vi "S2DS_ConfigReadWC (SubVI).vi"(0 "Refnum in":T3, 1 "WC Info list (in)":T1, 2 "Update present value?":bool, 3 "error in (no error)":errorcluster) -> (6 "Refnum out":T3, 7 "WC Info list (out)":T1, 9 "error out":errorcluster)   [LabVIEW 2025]
uses:
  <vilib>/Utility/config.llb/Config Data RefNum.ctl
  TYPE DEFS/S2DS_WC info.ctl
  TYPE DEFS/S2DS_Single WC info.ctl
  <vilib>/Utility/config.llb/Read Key (U32).vi
  <vilib>/Utility/config.llb/Read Key (String).vi
  <vilib>/Utility/config.llb/Read Key (Double).vi
  <vilib>/Utility/config.llb/NI_LVConfig.lvlib
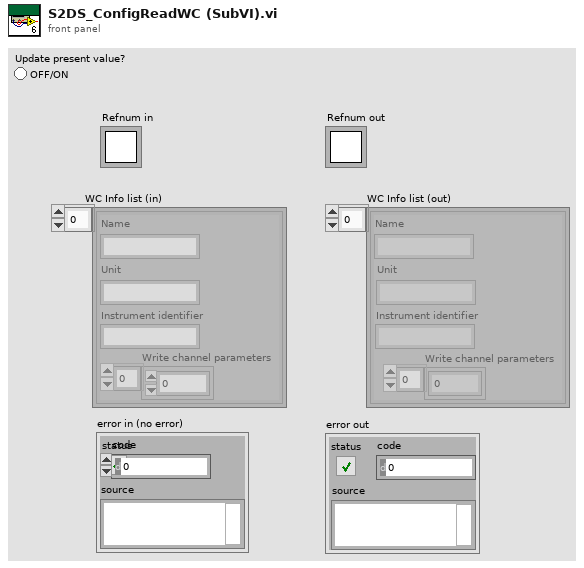
[diagram p1: front panel]
types:
  T1 = typedef "S2DS_WC info.ctl" = T2[]
  T2 = typedef "S2DS_Single WC info.ctl" = cluster{"Instrument identifier":string, "Write channel parameters":dbl[], "Name":string, "Unit":string}
  T3 = typedef "NI_LVConfig.lvlib/Config Data RefNum.ctl" = refnum<k1>
  T4 = cluster{"Instrument identifier":string, "Write channel parameters":dbl[], "Name":string, "Unit":string}
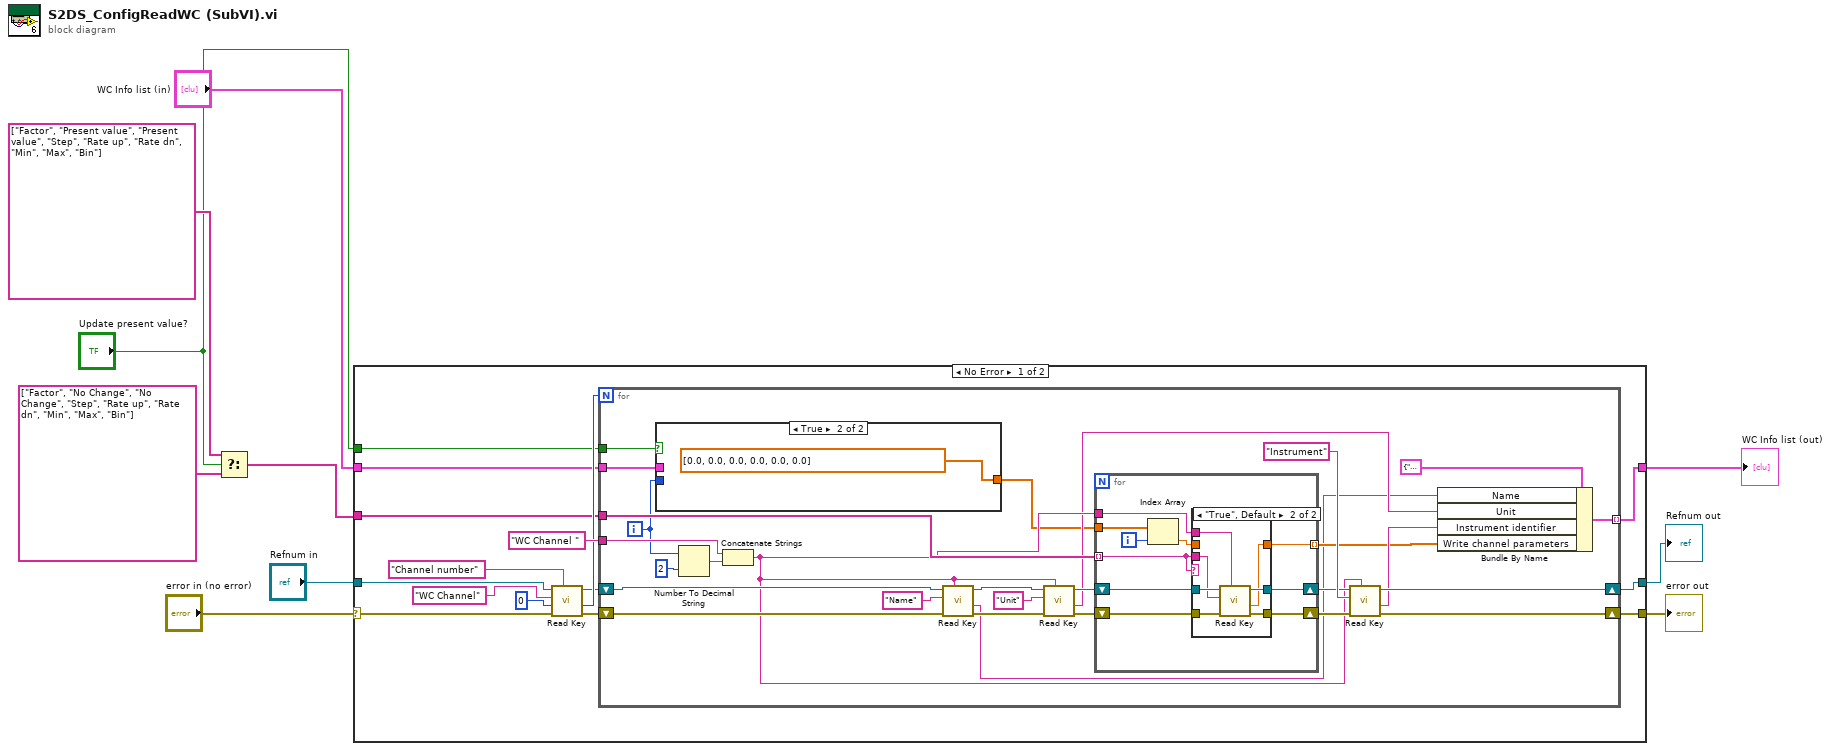
[diagram p0: block diagram]
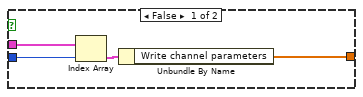
[diagram p2: hidden frame]
diagram:
  n1 = Select(t=string[] ["Factor", "Present value", "Present value", "Step", "Rate up", "Rate dn", "Min", "Max", "Bin"], s="Update present value?", f=string[] ["Factor", "No Change", "No Change", "Step", "Rate up", "Rate dn", "Min", "Max", "Bin"]) -> (s? t:f=w3:string[])
  n2 = case shown="No Error" "error in (no error)" {
    selector: "error in (no error)" -> [w15 w80]
    tunnel: [w25 w80] -> w10
    tunnel: [w24 w79] -> w9
    tunnel: [w22 w81] -> w8
    tunnel: "WC Info list (in)" -> [w12 w81]
    tunnel: "Refnum in" -> [w14 w79]
    tunnel: w3 -> [w13 _]
    tunnel: "Update present value?" -> [w11 _]
    frame No Error {
      n3 = call-poly <vilib>:"Read Key.vi"("section"="Channel number", "error in (no error)"=w15, "default value"=u32 0, "key"="WC Channel", "refnum"=w14) -> ("error out"=w16:errorcluster, "value"=w18:u32, "refnum out"=w17:T3)  [unwired: 4 out]
      n4 = for {
        N: w18 -> [_]
        shift-right: [w41] -> w24
        shift-left: w17 -> [w53]
        shift-right: [w40] -> w25
        shift-left: w16 -> [w52]
        tunnel: "WC Channel " -> [w49]
        tunnel: w13 -> [w39]
        tunnel: [w33] -> w22 mode=indexing
        tunnel: w12 -> [w29]
        tunnel: w11 -> [w26]
        i -> [w28]
        n5 = case shown="True" w26 {
          tunnel: w29 -> [w57 _]
          tunnel: w28 -> [w56 _]
          tunnel: [w54 dbl[] [0.0, 0.0, 0.0, 0.0, 0.0, 0.0] ("Write channel parameters")] -> w27
          frame False {
            n6 = Index Array(array=w57, index=w56) -> (element=w55:T2)
            n7 = Unbundle By Name(w55) -> ("Write channel parameters"=w54:dbl[])
          }
          frame True {
          }
        }
        n8 = Number To Decimal String(number=w28, width (-)=i16 2) -> (decimal integer string=w51:string)
        n9 = Concatenate Strings(w49, w51) -> (w36:string)
        n10 = call-poly <vilib>:"Read Key.vi"("section"=w36, "error in (no error)"=w52, "key"="Name", "refnum"=w53) -> ("error out"=w46:errorcluster, "value"=w30:string, "refnum out"=w47:T3)  [unwired: 2 in, 3 out]
        n11 = call-poly <vilib>:"Read Key.vi"("section"=w36, "error in (no error)"=w46, "key"="Unit", "refnum"=w47) -> ("error out"=w44:errorcluster, "value"=w31:string, "refnum out"=w43:T3)  [unwired: 2 in, 3 out]
        n12 = for {
          tunnel: w39 -> [w62] mode=indexing
          shift-right: [w67] -> w37
          shift-left: w43 -> [w68]
          shift-right: [w63] -> w38
          shift-left: w44 -> [w66]
          tunnel: w36 -> [w65]
          tunnel: [w64] -> w34 mode=indexing
          tunnel: w27 -> [w61]
          i -> [w60]
          n13 = Index Array(array=w61, index=w60) -> (element=w59:dbl)
          n14 = case shown="\"True\", Default" w62 {
            tunnel: w68 -> [w70 w78]
            tunnel: [w70 w77] -> w67
            tunnel: w66 -> [w71 w76]
            tunnel: w65 -> [_ w75]
            tunnel: w62 -> [_ w74]
            tunnel: [w69 w73] -> w64
            tunnel: [w71 w72] -> w63
            tunnel: w59 -> [w69 _]
            frame "No Change" {
            }
            frame "True", Default {
              n15 = call-poly <vilib>:"Read Key.vi"("section"=w75, "error in (no error)"=w76, "key"=w74, "refnum"=w78) -> ("error out"=w72:errorcluster, "value"=w73:dbl, "refnum out"=w77:T3)  [unwired: 1 in, 4 out]
            }
          }
        }
        n16 = call-poly <vilib>:"Read Key.vi"("section"=w36, "error in (no error)"=w38, "key"="Instrument", "refnum"=w37) -> ("error out"=w40:errorcluster, "value"=w35:string, "refnum out"=w41:T3)  [unwired: 2 in, 3 out]
        n17 = Bundle By Name(cluster=T4 {"Instrument identifier"="", "Write channel parameters"=[], "Name"="", "Unit"=""} ("Write channel info"), "Name"=w30, "Unit"=w31, "Instrument identifier"=w35, "Write channel parameters"=w34) -> (w33:T4)
      }
    }
    frame Error {
    }
  }
  "error out" <- w10
  "Refnum out" <- w9
  "WC Info list (out)" <- w8
